vi "Steuerung lesen.vi"(0 "Steuerung PNS Eingang":refnum<class "Steuerung PNS.lvclass">, 1 "Adressen":T1, 3 "error in (no error)":errorcluster caption="Fehler (Eingang, kein Fehler)") -> (7 "Steuerung PNS Ausgang":refnum<class "Steuerung PNS.lvclass">, 8 "Istwerte":u16[](array[numeric]), 10 "error out":errorcluster caption="Fehler (Ausgang)")   [LabVIEW 2020, in "Steuerung PNS.lvclass"]
doc: "Low Level Lesen der Steuerung mit den Adressen vom Input,\nIstwerte werden im Objekt gespeichert und als Output zur Verfügung gestellt.\nRIW"
uses:
  Steuerung PNS.lvclass
  Adresse.ctl
  Steuerung PNS.lvclass/Steuerung PNS.ctl
  <vilib>/NI/Modbus Library/API/Master/Modbus Master.lvclass
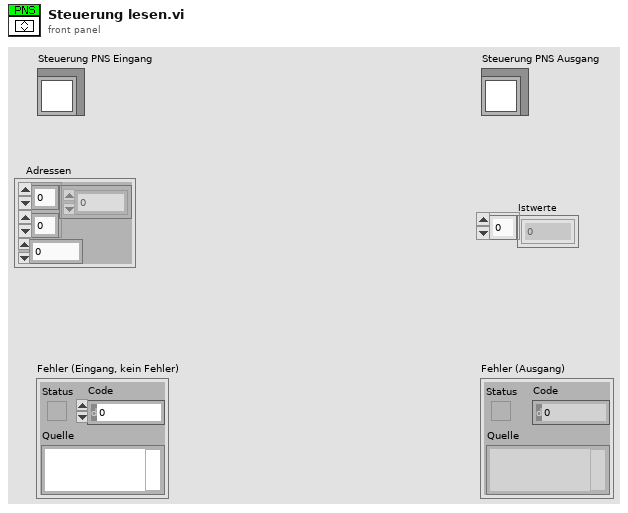
[diagram p1: front panel]
types:
  T1 = typedef "Steuerung PNS.lvclass/Adresse.ctl" = cluster{i32[][], i32}
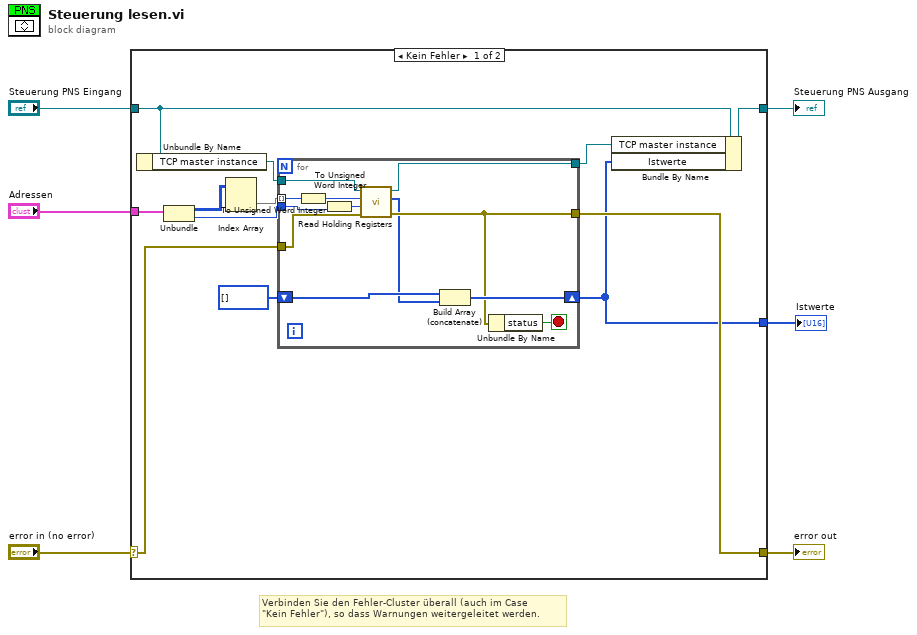
[diagram p0: block diagram]
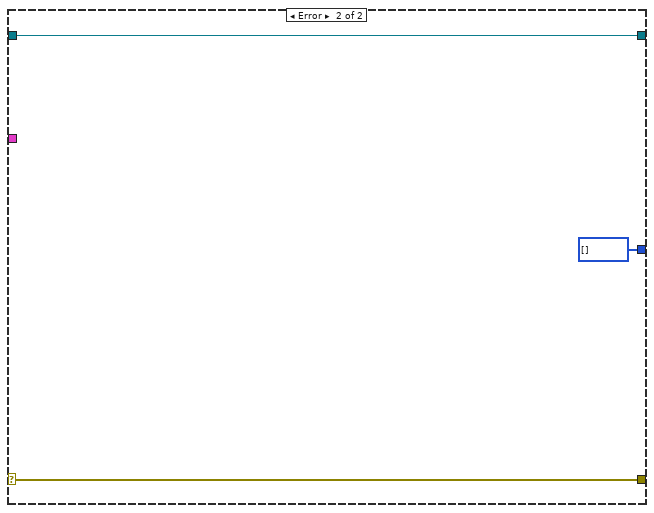
[diagram p2: hidden frame]
diagram:
  # "Verbinden Sie den Fehler-Cluster überall (auch im Case\n\"Kein Fehler\"), so dass Warnungen weitergeleitet werden."
  n1 = case shown="Kein Fehler" "error in (no error)" {
    selector: "error in (no error)" -> [w18 w33]
    tunnel: [w17 w33] -> w5
    tunnel: [w14 w32] -> w3
    tunnel: "Steuerung PNS Eingang" -> [w15 w32]
    tunnel: "Adressen" -> [w12 _]
    tunnel: [w8 u16[] []] -> w2
    frame No Error {
      n2 = Unbundle By Name(w15) -> ("TCP master instance"=w16:refnum<class "Modbus Master.lvclass">)
      n3 = Unbundle(w12) -> (w11:i32[][], w10:i32)
      n4 = Index Array(array=w11) -> (element=w9:i32[])  [unwired: 2 in]
      n5 = for {
        tunnel: w9 -> [w27] mode=indexing
        tunnel: [w23] -> w17
        tunnel: w18 -> [w22]
        tunnel: w10 -> [w26]
        shift-right: [w30] -> w8
        shift-left: u16[] [] -> [w29]
        tunnel: [w25] -> w13
        tunnel: w16 -> [w24]
        stop <- w28 stop-if-true
        n6 = To Unsigned Word Integer(number=w27) -> (unsigned 16bit integer=w21:u16)
        n7 = To Unsigned Word Integer(number=w26) -> (unsigned 16bit integer=w20:u16)
        n8 = call-dynamic "Read Holding Registers.vi"("error in"=w22, "number of inputs"=w20, "starting address"=w21, "Modbus master in"=w24) -> ("error out"=w23:errorcluster, "register values"=w19:u16[], "Modbus master out"=w25:refnum<class "Modbus Master.lvclass">)  [unwired: 5 in]
        n9 = Build Array (concatenate)(w29, w19) -> (w30:u16[])
        n10 = Unbundle By Name(w23) -> ("status"=w28:bool)
      }
      n11 = Bundle By Name(cluster=w15, "TCP master instance"=w13, "Istwerte"=w8) -> (w14:refnum<class "Steuerung PNS.lvclass">)
    }
    frame Error {
    }
  }
  "error out" <- w5
  "Steuerung PNS Ausgang" <- w3
  "Istwerte" <- w2
